vi "FTW-Ether-CreateEphemeralEndpoint.vi"(11 "error in":errorcluster) -> (4 "Ephemeral Endpoint":refnum<class "FTW-Endpoint.lvclass">, 6 "Actual Ephemeral Address":T1, 15 "error out":errorcluster)   [LabVIEW 2012, in "FTW-Actor.lvlib" / "FTW-Ether.lvclass"]
uses:
  FTW-Ether.lvclass
  Endpoint/FTW-Endpoint.lvclass
  Utility/FTW-Actor-Address.ctl
  FTW-Ether-MessageTransportScheme.ctl
  FTW-Ether-EndpointType.ctl
  FTW-Actor.lvlib
panel:
  # "Inputs"
  # "Outputs"
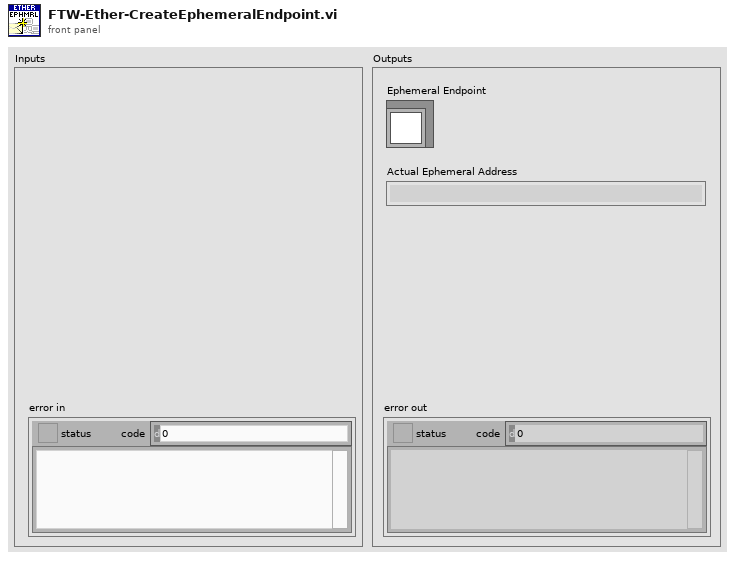
[diagram p1: front panel]
types:
  T1 = typedef "FTW-Actor.lvlib/FTW-Actor-Address.ctl" = string
  T2 = typedef "FTW-Actor.lvlib/FTW-Ether.lvclass/FTW-Ether-MessageTransportScheme.ctl" = enum16{"ØMQ TCP (tcp://)", "ØMQ In-Process (inproc://)", "LabVIEW Queues (lvq://)", "LabVIEW Network Streams (lvns://)"}
  T3 = typedef "FTW-Actor.lvlib/FTW-Ether.lvclass/FTW-Ether-EndpointType.ctl" = enum16{"Server", "Client", "Publisher", "Subscriber"}
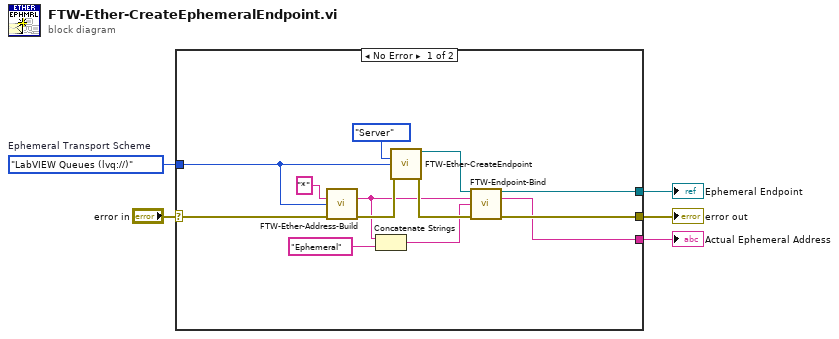
[diagram p0: block diagram]
diagram:
  w5 = FTW-Ether-MessageTransportScheme."LabVIEW Queues (lvq://)"  # Ephemeral Transport Scheme
  n1 = case shown="No Error" "error in" {
    selector: "error in" -> [w15 w19]
    tunnel: [w18 _] -> w1
    tunnel: [w17 w19] -> w2
    tunnel: w5 -> [w11 _]
    tunnel: [w16 _] -> w3
    frame No Error {
      n2 = call "FTW-Ether-Address-Build.vi"("Path"="*", "Message Transport Scheme"=w11, "error in"=w15) -> ("Endpoint Address"=w7:T1, "error out"=w10:errorcluster)  [unwired: 11 in]
      n3 = Concatenate Strings(w7, "Ephemeral" ("Requested Identity")) -> (w6:string)
      n4 = call "FTW-Ether-CreateEndpoint.vi"("Endpoint Type"=FTW-Ether-EndpointType."Server", "Message Transport Scheme"=w11, "error in"=w10) -> ("FTW Endpoint"=w14:refnum<class "FTW-Endpoint.lvclass">, "error out"=w12:errorcluster)  [unwired: 11 in]
      n5 = call-dynamic "FTW-Endpoint-Bind.vi"("FTW Endpoint"=w14, "Endpoint Address"=w7, "Requested Identity"=w6, "error in"=w12) -> ("FTW Endpoint out"=w18:refnum<class "FTW-Endpoint.lvclass">, "Actual Endpoint Address"=w16:T1, "error out"=w17:errorcluster)  [unwired: 8 in, 1 out]
    }
    frame Error {
    }
  }
  "error out" <- w2
  "Ephemeral Endpoint" <- w1
  "Actual Ephemeral Address" <- w3
